vi "Open Documentation.vi"(8 "error in (no error)":errorcluster, 10 "File Path":path) -> (0 "error out":errorcluster)   [LabVIEW 2021]
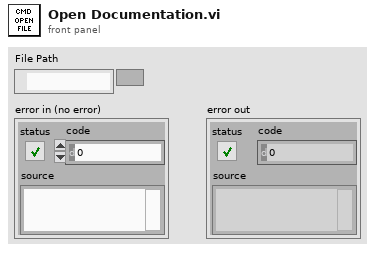
[diagram p1: front panel]
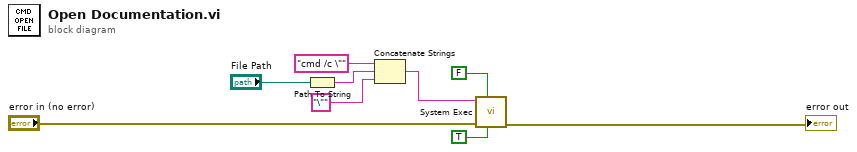
[diagram p0: block diagram]
diagram:
  n1 = Path To String(path="File Path") -> (string=w8:string)
  n2 = Concatenate Strings("cmd /c \"" ("string"), w8, "\"" ("string")) -> (w9:string)
  n3 = call <vilib>:"System Exec.vi"("run minimized? (F)"=TRUE, "wait until completion? (T)"=FALSE, "error in (no error)"="error in (no error)", "command line"=w9) -> ("error out"=→"error out":errorcluster)  [unwired: 4 in, 3 out]
